vi "KStoR.vi"(1 "K/S":dbl[](array[numeric])) -> (0 "Reflectance":dbl[](array[numeric]))   [LabVIEW 2013]
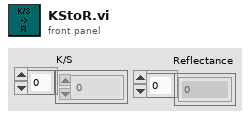
[diagram p1: front panel]
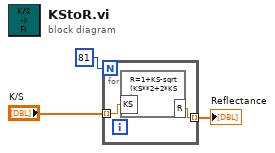
[diagram p0: block diagram]
diagram:
  n1 = for {
    N: 81 -> [_]
    tunnel: "K/S" -> [w5] mode=indexing
    tunnel: [w4] -> w1 mode=indexing
    n2 = formula code="R=1+KS-sqrt(KS**2+2*KS);"("KS"=w5) -> ("R"=w4:dbl)
  }
  "Reflectance" <- w1
